vi "Get real boat.vi"(2 "error in":errorcluster, 3 "Image":T1) -> (0 "error out":errorcluster, 1 "Matches":T2[](array[typedef]) {"Correlation Score" format="%.2f"; "Target Template Curve Score" format="%.2f"; "Template Target Curve Score" format="%.2f"; "Bounding Box"."y" format="%.2f"; "Bounding Box"."x" format="%.2f"; "Position"."y" format="%.2f"; "Position"."x" format="%.2f"; "Score" format="%.2f"; "Scale" format="%.2f"; "Angle" format="%.2f"; "Occlusion %" format="%.2f"})   [LabVIEW 2011]
uses:
  <vilib>/vision/Pattern Matching.llb/IMAQ GM Match Report.ctl
  <vilib>/vision/Image Controls.llb/IMAQ Image.ctl
  <vilib>/vision/Pattern Matching.llb/IMAQ Curve Parameters.ctl
  <vilib>/vision/Pattern Matching.llb/IMAQ Match Range Setting.ctl
  <vilib>/vision/NI_Vision_Development_Module.lvlib
panel:
  out "Templete Image":T1(plugin-control)
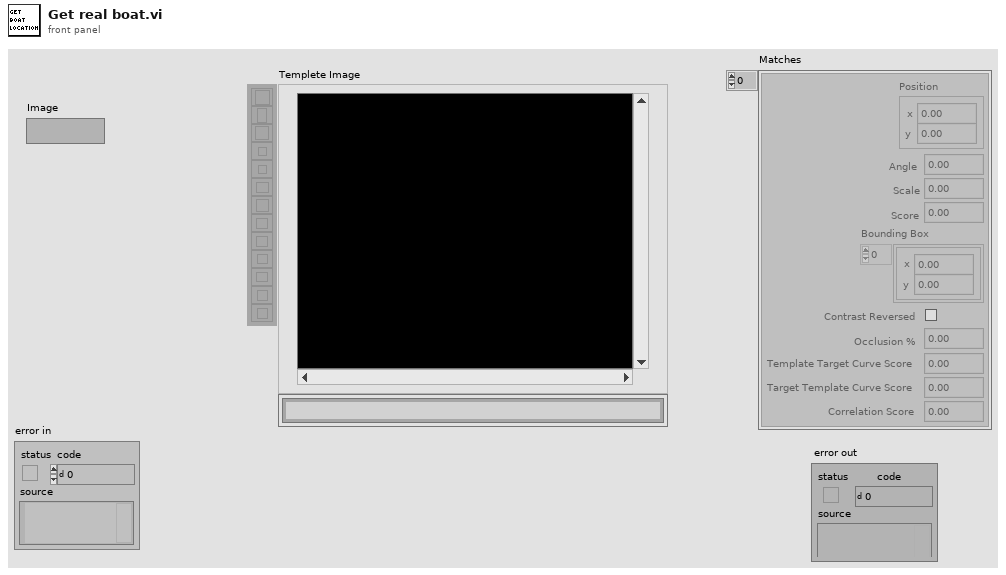
[diagram p1: front panel]
types:
  T1 = typedef "IMAQ Image.ctl" = refnum<image>
  T2 = typedef "IMAQ GM Match Report.ctl" = cluster{"Position":cluster{"x":sgl, "y":sgl}, "Angle":sgl, "Scale":sgl, "Score":sgl, "Bounding Box":cluster{"x":sgl, "y":sgl}[], "Contrast Reversed":bool, "Occlusion %":sgl, "Template Target Curve Score":sgl, "Target Template Curve Score":sgl, "Correlation Score":sgl}
  T3 = typedef "IMAQ Curve Parameters.ctl" = cluster{"Extraction Mode":u32, "Edge Threshold":i32, "Edge Filter Size":u32, "Min Length":i32, "Row Search Step Size":i32, "Col Search Step Size":i32, "Max Endpoint Gap":i32, "Closed":bool, "Subpixel":bool}
  T4 = typedef "IMAQ Match Range Setting.ctl" = cluster{"Match Constraints":u32, "Min":dbl, "Max":dbl}
  T5 = cluster{"Curve Parameters":T3, "Match Mode":cluster{"Rotation":bool, "Scale":bool, "Occlusion":bool, "Reserved":bool, "Reserved":bool, "Reserved":bool}, "Range Settings":T4[], "Number of Matches":i32, "Minimum Match Score":sgl, "SubPixel Accuracy":bool, "Adv. Geometric Match Options 2":cluster{"Setup Data Item":u16, "Item Value":dbl}[]}
  T6 = cluster{"Global Rectangle":i32[], "Contours":cluster{"ID":enum32{"External", "Internal"}, "Type":u32, "Coordinates":i32[]}[]}
  T7 = typedef "Image Type" = u32
  T8 = cluster{"histogram":u32[], "Minimal Value":sgl, "Maximal Value":sgl, "Starting Value":sgl, "Interval Width":sgl, "Mean Value":sgl, "Standard  Variation":sgl, "Area (pixels)":i32}
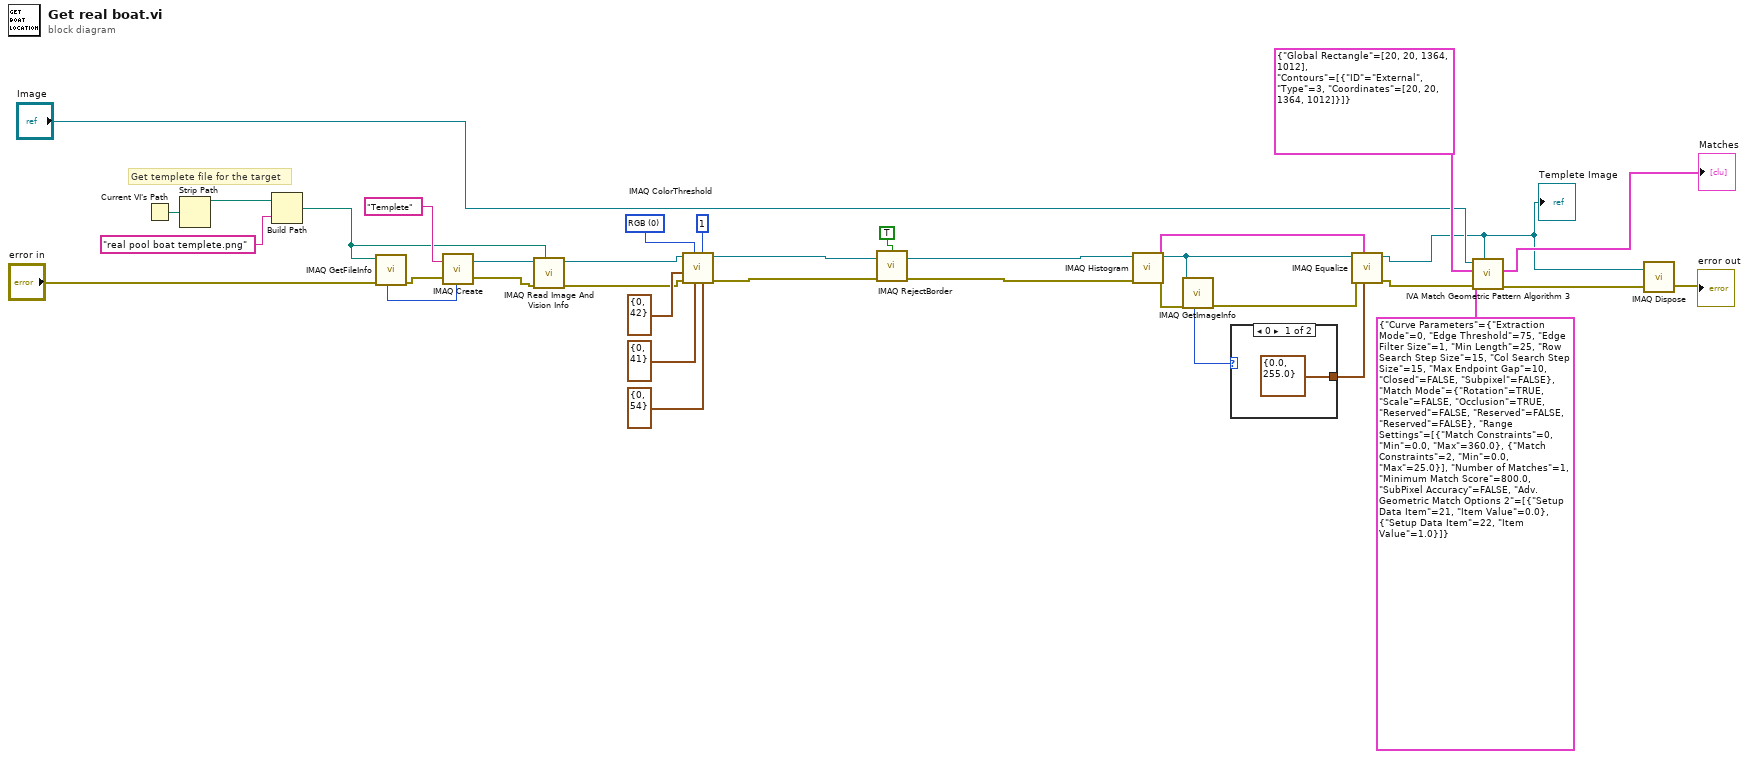
[diagram p0: block diagram]
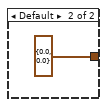
[diagram p2: hidden frame]
diagram:
  w18 = u16 0 items=["RGB", "HSL", "HSV", "HSI"] ("Color Mode")
  # "Get templete file for the target"
  n1 = Current VI's Path() -> (path=w31:path)
  n2 = Strip Path(path=w31) -> (stripped path=w30:path)  [unwired: 1 out]
  n3 = Build Path(base path=w30, name or relative path="real pool boat templete.png") -> (appended path=w26:path)
  n4 = call "IMAQ GetFileInfo"("error in (no error)"="error in", "File Path"=w26) -> ("error out"=w29:errorcluster, "Image Type"=w28:T7)  [unwired: 3 in, 5 out]
  n5 = call "IMAQ Create"("Image Name"="Templete", "Image Type"=w28, "error in (no error)"=w29) -> ("New Image"=w24:T1, "error out"=w25:errorcluster)  [unwired: 1 in, 1 out]
  n6 = call "IMAQ Read Image And Vision Info"("File Path"=w26, "error in (no error)"=w25, "Image"=w24) -> ("error out"=w2:errorcluster, "Image Out"=w4:T1)  [unwired: 1 in, 6 out]
  n7 = call "IMAQ ColorThreshold"("Blue or Luma or Val or Inten Range"=cluster{"Lower value":i32, "Upper value":i32} {"Lower value"=0, "Upper value"=54}, "Replace Value"=1, "Green or Sat Range"=cluster{"Lower value":i32, "Upper value":i32} {"Lower value"=0, "Upper value"=41}, "Color Mode"=w18, "error in (no error)"=w2, "Red or Hue Range"=cluster{"Lower value":i32, "Upper value":i32} {"Lower value"=0, "Upper value"=42}, "Image Src"=w4) -> ("error out"=w14:errorcluster, "Image Dst Out"=w12:T1)  [unwired: 1 in, 2 out]
  n8 = call "IMAQ RejectBorder"("error in (no error)"=w14, "Image Src"=w12, "Connectivity 4/8 (8)"=TRUE) -> ("error out"=w11:errorcluster, "Image Dst Out"=w8:T1)  [unwired: 1 in, 2 out]
  n9 = call "IMAQ Histogram"("error in (no error)"=w11, "Image"=w8) -> ("error out"=w7:errorcluster, "Histogram Report"=w10:T8)  [unwired: 3 in, 5 out]
  n10 = call "IMAQ GetImageInfo"("error in (no error)"=w7, "Image"=w8) -> ("error out"=w6:errorcluster, "Image Type"=w9:T7)  [unwired: 8 out]
  n11 = case shown="0" w9 {
    tunnel: [cluster{"Minimum":sgl, "Maximum":sgl} {"Minimum"=0.0, "Maximum"=255.0} ("Range") cluster{"Minimum":sgl, "Maximum":sgl} {"Minimum"=0.0, "Maximum"=0.0} ("Range")] -> w5
    frame 0 {
    }
    frame Default {
    }
  }
  n12 = call "IMAQ Equalize"("Range"=w5, "Histogram Report"=w10, "error in (no error)"=w6, "Image Src"=w8) -> ("error out"=w1:errorcluster, "Image Dst Out"=w3:T1)  [unwired: 2 in, 4 out]
  "Templete Image" <- w3
  n13 = call <vilib>:"IVA Match Geometric Pattern Algorithm 3.vi"("Template"=w3, "error in (no error)"=w1, "Settings"=T5 {"Curve Parameters"={"Extraction Mode"=0, "Edge Threshold"=75, "Edge Filter Size"=1, "Min Length"=25, "Row Search Step Size"=15, "Col Search Step Size"=15, "Max Endpoint Gap"=10, "Closed"=FALSE, "Subpixel"=FALSE}, "Match Mode"={"Rotation"=TRUE, "Scale"=FALSE, "Occlusion"=TRUE, "Reserved"=FALSE, "Reserved"=FALSE, "Reserved"=FALSE}, "Range Settings"=[{"Match Constraints"=0, "Min"=0.0, "Max"=360.0}, {"Match Constraints"=2, "Min"=0.0, "Max"=25.0}], "Number of Matches"=1, "Minimum Match Score"=800.0, "SubPixel Accuracy"=FALSE, "Adv. Geometric Match Options 2"=[{"Setup Data Item"=21, "Item Value"=0.0}, {"Setup Data Item"=22, "Item Value"=1.0}]} ("Settings (Geometric Matching 1)"), "ROI Descriptor"=T6 {"Global Rectangle"=[20, 20, 1364, 1012], "Contours"=[{"ID"=enum."External", "Type"=3, "Coordinates"=[20, 20, 1364, 1012]}]} ("ROI Descriptor (Geometric Matching 1)"), "Image"="Image") -> ("error out"=w22:errorcluster, "Matches"=→"Matches":T2[])  [unwired: 5 out]
  n14 = call "IMAQ Dispose"("Image"=w3, "error in (no error)"=w22) -> ("error out"=→"error out":errorcluster)  [unwired: 4 in]
